vi "Pre-Init.vi"(8 "error in (no error)":errorcluster, 11 "Simple VISA Reader Driver in":refnum<class "Simple VISA Reader Driver.lvclass">) -> (0 "error out":errorcluster, 3 "Simple VISA Reader Driver out":refnum<class "Simple VISA Reader Driver.lvclass">)   [LabVIEW 2019, in "Simple VISA Reader Driver.lvclass"]
uses:
  Simple VISA Reader Driver.lvclass
  C:/GitHub/NHMFL_Core/Libraries/Instruments/Instrument Driver/Instrument Driver.lvclass
  Instrument Driver/Instrument Driver.lvclass/Instrument Driver.ctl
  Instrument Driver/Write Timing group name.vi
  VISA Instrument/VISA Instrument.lvclass
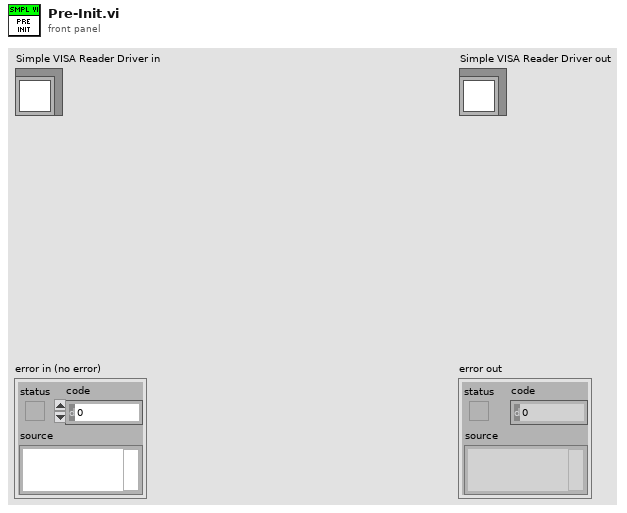
[diagram p1: front panel]
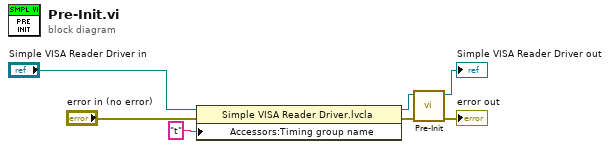
[diagram p0: block diagram]
diagram:
  n1 = property class="Simple VISA Reader Driver.lvcla"(reference="Simple VISA Reader Driver in", error in="error in (no error)", "Accessors:Timing group name"="t" ("Timing group name")) -> (reference out=w2:refnum<class "Simple VISA Reader Driver.lvclass">, error out=w4:errorcluster)
  n2 = call-parent "Pre-Init.vi"("error in (no error)"=w4, "Instrument Driver in"=w2) -> ("error out"=→"error out":errorcluster, "Instrument Driver out"=→"Simple VISA Reader Driver out":refnum<class "Simple VISA Reader Driver.lvclass">)  [unwired: 8 in]
